vi "Clean Up FP.vi"(8 "error in (no error)":errorcluster, 11 "vi ref in":refnum<vi>) -> (0 "error out":errorcluster, 3 "vi ref out":refnum<vi>)   [LabVIEW 2021]
uses:
  <vilib>/Utility/miscctls.llb/LVPositionTypeDef.ctl
panel:
  # "This VI cleans up the Front Panel of the scripted\nSubVI by applying standard placement rules"
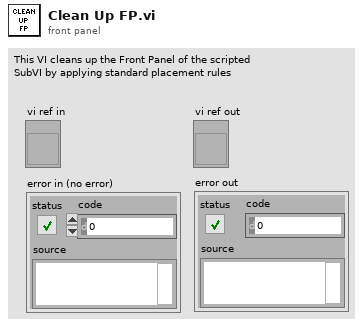
[diagram p1: front panel]
types:
  T1 = enum32{"Invalid", "Standard", "Closed", "Hidden", "Minimized", "Maximized"}
  T2 = typedef "LVPositionTypeDef.ctl" = cluster{"Left":i32, "Top":i32}
  T3 = typedef "LVRectTypeDef.ctl" = cluster{"Left":i16, "Top":i16, "Right":i16, "Bottom":i16}
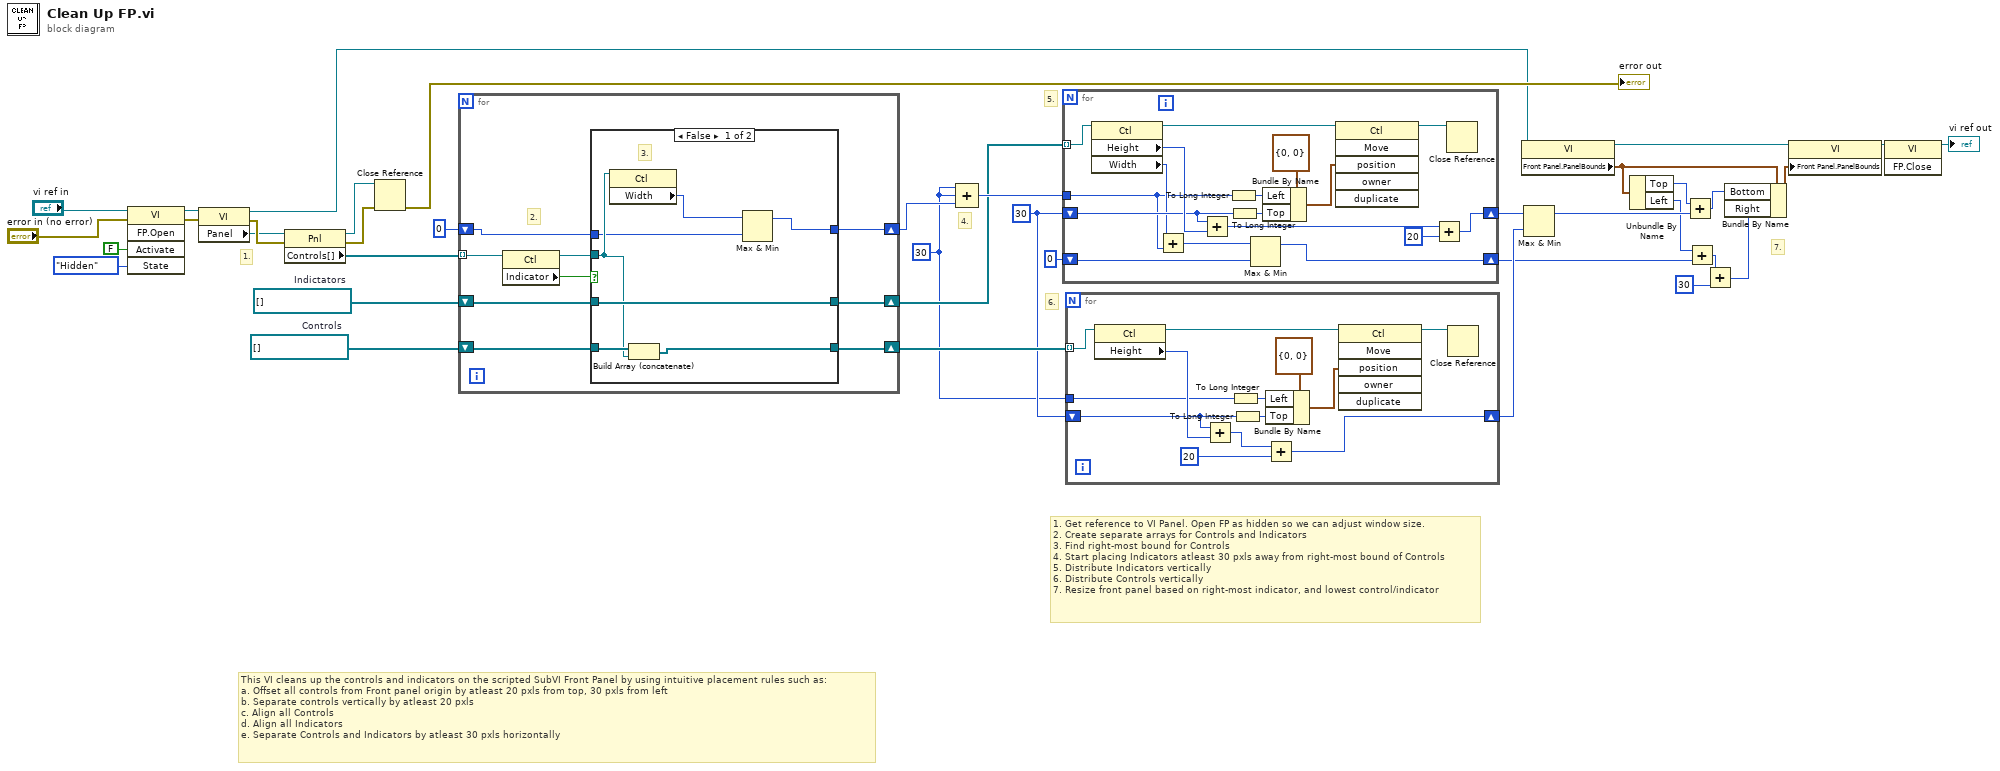
[diagram p0: block diagram]
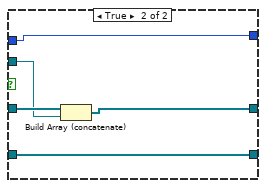
[diagram p2: hidden frame]
diagram:
  w28 = u32 30 ("Left")
  w29 = u32 30
  w36 = refnum<vi>[] []  # Indictators
  w37 = refnum<vi>[] []  # Controls
  # "7."
  # "This VI cleans up the controls and indicators on the scripted SubVI Front Panel by using intuitive placement rules such as:\na. Offset all controls from Front panel origin by atleast 20 pxls from top, 30 pxls from left\nb. Separate controls vertically by atleast 20 pxls\nc. Align all Controls\nd. Align all Indicators\ne. Separate Controls and Indicators by atleast 30 pxls horizontally"
  # "1. Get reference to VI Panel. Open FP as hidden so we can adjust window size.\n2. Create separate arrays for Controls and Indicators\n3. Find right-most bound for Controls\n4. Start placing Indicators atleast 30 pxls away from right-most bound of Controls\n5. Distribute Indicators vertically\n6. Distribute Controls vertically\n7. Resize front panel based on right-most indicator, and lowest control/indicator"
  # "6."
  # "5."
  # "4."
  # "1."
  n1 = invoke class="VI" method="FP.Open"(reference="vi ref in", error in="error in (no error)", "Activate"=FALSE ("Activate?"), "State"=T1."Hidden") -> (reference out=w10:refnum<vi>, error out=w6:errorcluster)  [unwired: 1 in, 3 out]
  n2 = property class="VI"(reference=w10, error in=w6) -> (reference out=w23:refnum<vi>, error out=w27:errorcluster, "Panel"=w24:refnum<vi>)
  n3 = property class="Pnl"(reference=w24, error in=w27) -> (reference out=w31:refnum<vi>, error out=w26:errorcluster, "Controls[]"=w38:refnum<vi>[])
  n4 = Close Reference(reference=w31, error in (no error)=w26) -> (error out=→"error out":errorcluster)
  n5 = for {
    tunnel: w38 -> [w39] mode=indexing
    shift-right: [w42] -> w32
    shift-left: w37 -> [w46]
    shift-right: [w43] -> w33
    shift-left: w36 -> [w45]
    shift-right: [w40] -> w30
    shift-left: u32 0 ("right") -> [w41]
    # "2."
    n6 = property class="Ctl"(reference=w39) -> (reference out=w44:refnum<vi>, "Indicator"=w47:bool)  [unwired: 1 in, 1 out]
    n7 = case shown="False" w47 {
      tunnel: w46 -> [w54 w56]
      tunnel: w45 -> [w52 w59]
      tunnel: w44 -> [w51 w58]
      tunnel: [w52 w57] -> w43
      tunnel: [w53 w56] -> w42
      tunnel: w41 -> [w49 w55]
      tunnel: [w48 w55] -> w40
      frame False {
        # "3."
        n8 = property class="Ctl"(reference=w51) -> ("Width"=w50:u32)  [unwired: 1 in, 2 out]
        n9 = Build Array (concatenate)(w54, w51) -> (w53:refnum<vi>[])
        n10 = Max & Min(x=w50, y=w49) -> (max(x,y)=w48:u32)  [unwired: 1 out]
      }
      frame True {
        n11 = Build Array (concatenate)(w59, w58) -> (w57:refnum<vi>[])
      }
    }
  }
  n12 = Compound Arithmetic op=ADD(w28, w28, w30) -> (w34:u32)
  n13 = for {
    shift-right: [w72] -> w22
    shift-left: w29 -> [w67]
    tunnel: w34 -> [w61]
    tunnel: w33 -> [w69] mode=indexing
    shift-right: [w63] -> w5
    shift-left: u32 0 -> [w64]
    n14 = property class="Ctl"(reference=w69) -> (reference out=w75:refnum<vi>, "Height"=w71:u32, "Width"=w62:u32)  [unwired: 1 in, 1 out]
    n15 = Add(x=w62, y=w61) -> (x+y=w60:u32)
    n16 = Add(x=w67, y=w71) -> (x+y=w70:u32)
    n17 = To Long Integer(number=w61) -> (32bit integer=w65:i32)
    n18 = To Long Integer(number=w67) -> (32bit integer=w68:i32)
    n19 = Max & Min(x=w60, y=w64) -> (max(x,y)=w63:u32)  [unwired: 1 out]
    n20 = Bundle By Name(cluster=T2 {"Left"=0, "Top"=0} ("position"), "Left"=w65, "Top"=w68) -> (w73:T2)
    n21 = invoke class="Ctl" method="Move"(reference=w75, "position"=w73) -> (reference out=w66:refnum<vi>)  [unwired: 4 in, 5 out]
    n22 = Add(x=w70, y=u32 20) -> (x+y=w72:u32)
    n23 = Close Reference(reference=w66) -> ()  [unwired: 1 in, 1 out]
  }
  n24 = for {
    shift-right: [w85] -> w21
    shift-left: w29 -> [w80]
    tunnel: w32 -> [w82] mode=indexing
    tunnel: w28 -> [w77]
    n25 = property class="Ctl"(reference=w82) -> (reference out=w88:refnum<vi>, "Height"=w84:u32)  [unwired: 1 in, 1 out]
    n26 = Add(x=w80, y=w84) -> (x+y=w83:u32)
    n27 = To Long Integer(number=w77) -> (32bit integer=w78:i32)
    n28 = To Long Integer(number=w80) -> (32bit integer=w81:i32)
    n29 = Bundle By Name(cluster=T2 {"Left"=0, "Top"=0} ("position"), "Left"=w78, "Top"=w81) -> (w86:T2)
    n30 = Add(x=w83, y=u32 20) -> (x+y=w85:u32)
    n31 = invoke class="Ctl" method="Move"(reference=w88, "position"=w86) -> (reference out=w79:refnum<vi>)  [unwired: 4 in, 5 out]
    n32 = Close Reference(reference=w79) -> ()  [unwired: 1 in, 1 out]
  }
  n33 = property class="VI"(reference=w23) -> (reference out=w18:refnum<vi>, "Front Panel.PanelBounds"=w17:T3)  [unwired: 1 in, 1 out]
  n34 = Max & Min(x=w22, y=w21) -> (max(x,y)=w19:u32)  [unwired: 1 out]
  n35 = Unbundle By Name(w17) -> ("Top"=w20:i16, "Left"=w12:i16)
  n36 = Add(x=w20, y=w19) -> (x+y=w13:u32)
  n37 = Add(x=w12, y=w5) -> (x+y=w4:u32)
  n38 = Add(x=w4, y=u32 30 ("Left")) -> (x+y=w2:u32)
  n39 = Bundle By Name(cluster=w17, "Bottom"=w13, "Right"=w2) -> (w16:T3)
  n40 = property class="VI"(reference=w18, "Front Panel.PanelBounds"=w16) -> (reference out=w15:refnum<vi>)  [unwired: 1 in, 1 out]
  n41 = invoke class="VI" method="FP.Close"(reference=w15) -> (reference out=→"vi ref out":refnum<vi>)  [unwired: 2 in, 2 out]
